vi "Monitor - Status.vi"(0 "VISA Refnum in":refnum<visa-resource-name>, 11 "Error In":errorcluster) -> (4 "VISA Refnum out":refnum<visa-resource-name>, 6 "Output Status":T1, 15 "Error Out":errorcluster)   [LabVIEW 2025]
panel:
  out "return count":u32
  out "Command":string
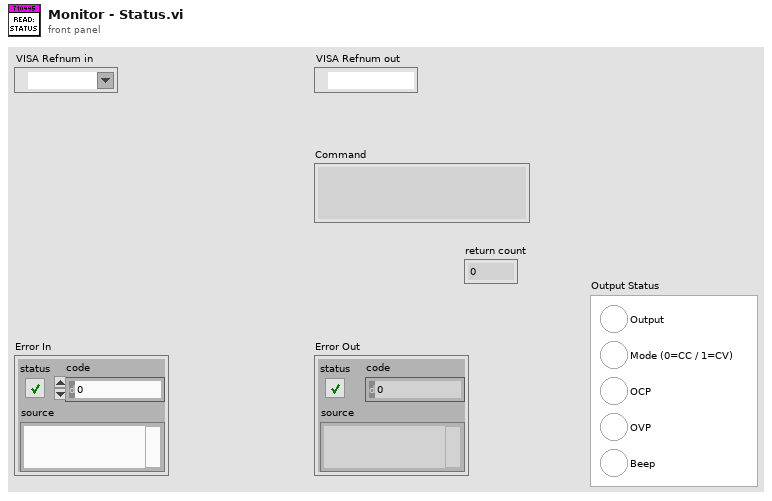
[diagram p1: front panel]
types:
  T1 = cluster{"Output":bool, "Mode (0=CC / 1=CV)":bool, "OCP":bool, "OVP":bool, "Beep":bool}
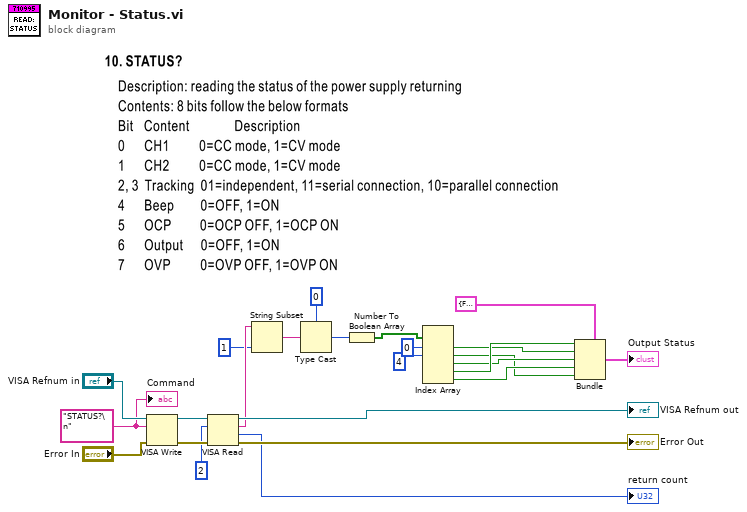
[diagram p0: block diagram]
diagram:
  w18 = "STATUS?\n"
  n1 = VISA Write(VISA resource name="VISA Refnum in", write buffer=w18, error in (no error)="Error In") -> (VISA resource name out=w20:refnum<visa-resource-name>, error out=w21:errorcluster)  [unwired: 1 out]
  n2 = VISA Read(VISA resource name=w20, byte count=u32 2, error in (no error)=w21) -> (VISA resource name out=→"VISA Refnum out":refnum<visa-resource-name>, read buffer=w15:string, return count=→"return count":u32, error out=→"Error Out":errorcluster)
  n3 = String Subset(string=w15, length (rest)=1 ("length (rest)")) -> (substring=w13:string)  [unwired: 1 in]
  n4 = Type Cast(type=u8 0 ("default (0 I32)"), x=w13) -> (*(type *) &x=w11:u8)
  n5 = Number To Boolean Array(number=w11) -> (Boolean array=w10:bool[])
  n6 = Index Array(array=w10, index #1=0 ("index"), index #2=4 ("index")) -> (element #1=w5:bool, element #2=w2:bool, element #3=w4:bool, element #4=w6:bool, element #5=w3:bool)  [unwired: 3 in]
  n7 = Bundle(cluster=T1 {"Output"=FALSE, "Mode (0=CC / 1=CV)"=FALSE, "OCP"=FALSE, "OVP"=FALSE, "Beep"=FALSE} ("Output Status"), "Output"=w6, "Mode (0=CC / 1=CV)"=w5, "OCP"=w4, "OVP"=w3, "Beep"=w2) -> (→"Output Status":T1)
  "Command" <- w18
